vi "TEST Search Replace Query.vi"() -> ()   [LabVIEW 2013, in "Carya Config.lvclass"]
doc: "Copyright 2018, Carya Automatisering, Wiebe Walstra."
uses:
  Carya Config.lvclass
  CConfig Object/Search Replace Query/Search Replace Query.lvclass
panel:
  in  "String 3":string="\n[one]\nkey=this is only a test\n\n[two]\nkey=this is only a test\narray0=0,1,2,3,4,5,6,7,8\narray1=\narray2=0,1,2"
  out "String":string
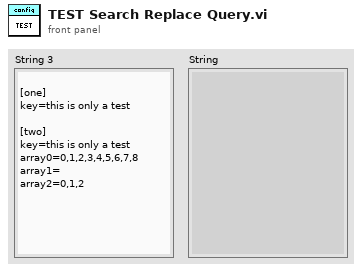
[diagram p1: front panel]
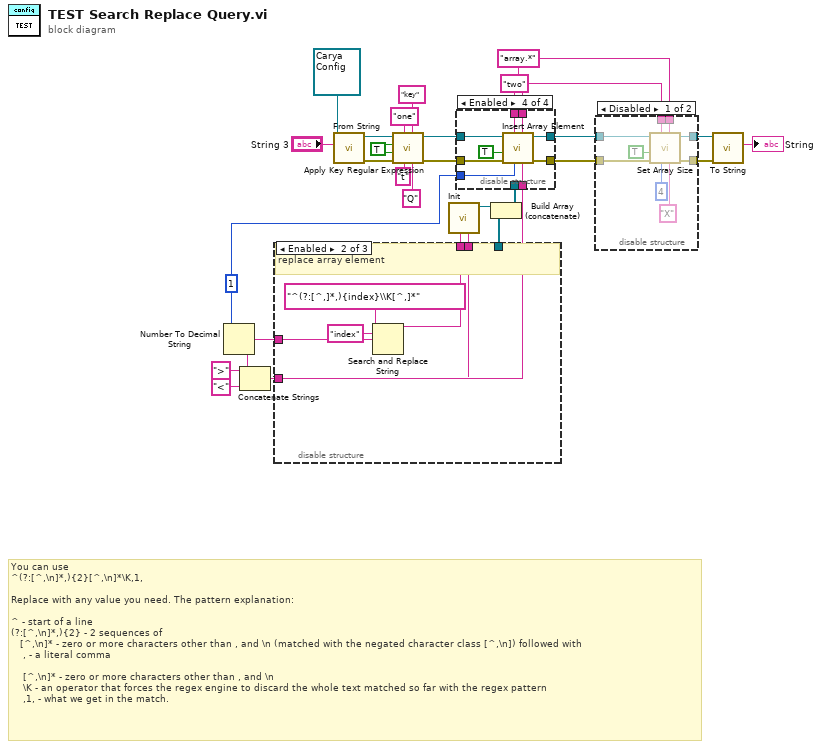
[diagram p0: block diagram]
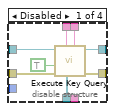
[diagram p3: hidden frame]
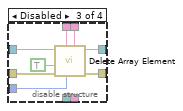
[diagram p5: hidden frame]
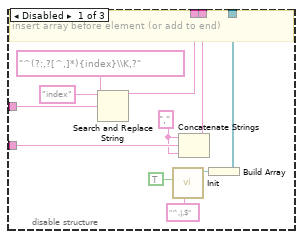
[diagram p6: hidden frame]
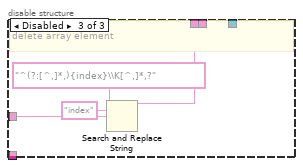
[diagram p7: hidden frame]
diagram:
  w1 = "array.*" ("Key name")
  w2 = "two" ("Section name")
  w7 = 1 ("number")
  w17 = TRUE ("Replace all? [F]")
  # "You can use\n^(?:[^,\\n]*,){2}[^,\\n]*\\K,1,\n\nReplace with any value you need. The pattern explanation:\n\n^ - start of a line\n(?:[^,\\n]*,){2} - 2 sequences of \n   [^,\\n]* - zero or more characters other than , and \\n (matched with the negated character class [^,\\n]) followed with\n    , - a literal comma\n\n    [^,\\n]* - zero or more characters other than , and \\n \n    \\K - an operator that forces the regex engine to discard the whole text matched so far with the regex pattern\n    ,1, - what we get in the match."
  n1 = Number To Decimal String(number=w7) -> (decimal integer string=w12:string)  [unwired: 1 in]
  n2 = Concatenate Strings(">" ("string"), w12, "<" ("string")) -> (w6:string)
  n3 = disable-structure shown="Enabled" {
    disable-tunnel: [w38 w43 w47] -> w16
    disable-tunnel: [w36 w40 _] -> w15
    disable-tunnel: w12 -> [w35 w41 w45]
    disable-tunnel: w6 -> [w34 w40 _]
    disable-tunnel: [w30 _ _] -> w11
    frame Disabled {
      w29 = "," ("f")
      # "insert array before element (or add to end)"
      n4 = Search and Replace String(input string="^(?:,?[^,]*){index}\\K,?" ("Regex"), search string="index", replace string=w35) -> (result string=w38:string)  [unwired: 5 in, 3 out]
      n5 = call "Init.vi"("Search"="^,|,$" ("Regex"), "Replace all? [F]"=TRUE) -> ("Find First Query out"=w31:refnum<class "Search Replace Query.lvclass">)  [unwired: 8 in, 1 out]
      n6 = Concatenate Strings(w29, w34, w29) -> (w36:string)
      n7 = Build Array(w31) -> (w30:refnum<class "Search Replace Query.lvclass">[])
    }
    frame Enabled {
      # "replace array element"
      n8 = Search and Replace String(input string="^(?:[^,]*,){index}\\K[^,]*" ("Regex"), search string="index", replace string=w41) -> (result string=w43:string)  [unwired: 5 in, 3 out]
    }
    frame Disabled {
      # "delete array element"
      n9 = Search and Replace String(input string="^(?:[^,]*,){index}\\K[^,]*,?" ("Regex"), search string="index", replace string=w45) -> (result string=w47:string)  [unwired: 5 in, 3 out]
    }
  }
  n10 = call-dynamic "From String.vi"("String"="String 3", "Carya Config in"=refnum<class "Carya Config.lvclass"> refnum) -> ("error out"=w26:errorcluster, "Carya Config out"=w24:refnum<class "Carya Config.lvclass">)  [unwired: 7 in, 1 out]
  n11 = call-dynamic "Apply Key Regular Expression.vi"("Replace"="Q", "Key name"="key", "Regex"="t", "Section name"="one", "error in (no error)"=w26, "RegEx? search [T]"=w17, "Replace all? [F]"=w17, "Carya Config in"=w24) -> ("error out"=w25:errorcluster, "Carya Config out"=w18:refnum<class "Carya Config.lvclass">)  [unwired: 2 in]
  n12 = call "Init.vi"("Replace"=w15, "Search"=w16) -> ("Find First Query out"=w10:refnum<class "Search Replace Query.lvclass">)  [unwired: 8 in, 1 out]
  n13 = Build Array (concatenate)(w10, w11) -> (w9:refnum<class "Search Replace Query.lvclass">[])
  n14 = disable-structure shown="Enabled" {
    disable-tunnel: w25 -> [w56 w57 w66 w75]
    disable-tunnel: [w55 w57 w65 w74] -> w19
    disable-tunnel: w18 -> [w54 w58 w64 w73]
    disable-tunnel: [w53 w58 w63 w72] -> w4
    disable-tunnel: w2 -> [w52 _ w61 w70]
    disable-tunnel: w1 -> [w51 _ w62 w71]
    disable-tunnel: w9 -> [w50 _ _ _]
    disable-tunnel: w7 -> [_ _ w60 w69]
    disable-tunnel: w6 -> [_ _ _ w67]
    frame Disabled {
      n15 = call-dynamic "Execute Key Query.vi"("Key name"=w51, "Key queries"=w50, "Section name"=w52, "error in (no error)"=w56, "Use Key Regex? [F]"=TRUE, "Carya Config in"=w54) -> ("error out"=w55:errorcluster, "Carya Config out"=w53:refnum<class "Carya Config.lvclass">)  [unwired: 3 in, 1 out]
    }
    frame Disabled {
    }
    frame Disabled {
      n16 = call-dynamic "Delete Array Element.vi"("Key name"=w62, "Index"=w60, "Section name"=w61, "error in (no error)"=w66, "Use Key Regex? [F]"=TRUE, "Carya Config in"=w64) -> ("error out"=w65:errorcluster, "Carya Config out"=w63:refnum<class "Carya Config.lvclass">)  [unwired: 4 in]
    }
    frame Enabled {
      n17 = call-dynamic "Insert Array Element.vi"("Insert"=w67, "Key name"=w71, "Index"=w69, "Section name"=w70, "error in (no error)"=w75, "Use Key Regex? [F]"=TRUE, "Carya Config in"=w73) -> ("error out"=w74:errorcluster, "Carya Config out"=w72:refnum<class "Carya Config.lvclass">)  [unwired: 3 in]
    }
  }
  n18 = disable-structure shown="Disabled" {
    disable-tunnel: w19 -> [w84 w85]
    disable-tunnel: [w83 w85] -> w5
    disable-tunnel: w4 -> [w82 w86]
    disable-tunnel: [w81 w86] -> w3
    disable-tunnel: w2 -> [w80 _]
    disable-tunnel: w1 -> [w79 _]
    frame Disabled {
      n19 = call-dynamic "Set Array Size.vi"("Default"="X", "Key name"=w79, "Index"=4, "Section name"=w80, "error in (no error)"=w84, "Use Key Regex? [F]"=TRUE, "Carya Config in"=w82) -> ("error out"=w83:errorcluster, "Carya Config out"=w81:refnum<class "Carya Config.lvclass">)  [unwired: 3 in]
    }
    frame Enabled {
    }
  }
  n20 = call-dynamic "To String.vi"("error in (no error)"=w5, "Carya Config in"=w3) -> ("String"=→"String":string)  [unwired: 7 in, 2 out]
